vi "Process.vi"(0 "reference in":refnum<class "Grapher.lvclass">, 5 "error in":errorcluster) -> (14 "reference out":refnum<class "Grapher.lvclass">, 19 "error out":errorcluster)   [LabVIEW 2023, in "Grapher.lvclass"]
uses:
  Grapher.lvclass
  Grapher.lvclass/Grapher.ctl
  <vilib>/Utility/SystemLogging/NI_SystemLogging.lvlib
  Types/Indicators.ctl
  builds/PowerModuleInterface/PowerModuleInterface.lvlibp/Classes/PowerModule_interface/PowerModuleInterface.lvclass
panel:
  out "error info":errorcluster
  out "Last Command":string
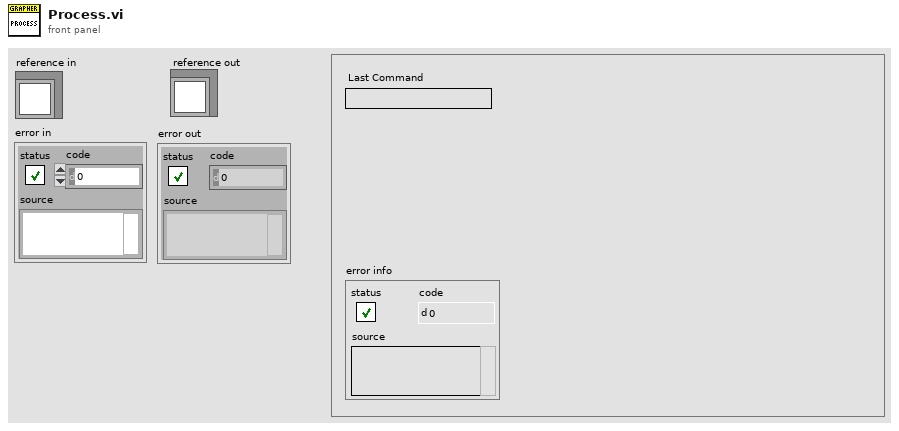
[diagram p1: front panel]
types:
  T1 = typedef "Indicators.ctl" = cluster{"XY Graph":refnum<vi>, "Mini Chart":refnum<vi>, "Voltage":refnum<vi>, "Current":refnum<vi>, "Power":refnum<vi>, "Function":refnum<vi>, "Charging":refnum<vi>, "Discharging":refnum<vi>}
  T2 = cluster{"Core":cluster{"Timeout":i32, "Events":cluster{"EventsToProcess":refnum<event-registration>}, "EventFromProcess":refnum<user-event>, "ProcessSyncQueue":refnum<queue>, "QueueFromProcess":refnum<queue>, "Command":string, "Data":variant}, "Chart History":cluster{"local timestamp":dbl[], "system timestamp":dbl[], "measured voltage":dbl[], "measured current":dbl[], "setpoint voltage":dbl[], "setpoint current":dbl[]}, "Use Local Time?":bool, "Graph Samples":u32, "Graph Decimation":i32, "Indicator Refs":T1, "Pause?":bool, "Power Module":refnum<class "PowerModuleInterface.lvclass">}
  T3 = cluster{"local timestamp":dbl[], "system timestamp":dbl[], "measured voltage":dbl[], "measured current":dbl[], "setpoint voltage":dbl[], "setpoint current":dbl[]}
  T4 = enum32{"Invalid", "Standard", "Closed", "Hidden", "Minimized", "Maximized"}
  T5 = cluster{"EventsToProcess":refnum<event-registration>}
  T6 = typedef "PowerModuleInterface.lvlibp/PowerModuleInterface.lvclass/Measurements.ctl" = cluster{"measured voltage (V)":dbl, "measured current (A)":dbl, "setpoint voltage (V)":dbl, "setpoint current (A)":dbl, "timestamp":dbl}
  T7 = typedef "Power Function.ctl" = enum16{"REGEN (LOAD)", "STANDBY", "SUPPLY (SOURCE)"}
  T8 = cluster{"system timestamp":dbl[], "measured voltage":dbl[]}
  T9 = cluster{"system timestamp":dbl[], "setpoint voltage":dbl[]}
  T10 = cluster{"system timestamp":dbl[], "measured current":dbl[]}
  T11 = cluster{"system timestamp":dbl[], "setpoint current":dbl[]}
  T12 = cluster{"system timestamp":dbl[], "setpoint current":dbl[]}[]
  T13 = typedef "Grapher.lvclass/ObjectAttributes.ctl" = cluster{"Indicator Refs":T1, "Update Rate (ms)":i32, "Power Module":refnum<class "PowerModuleInterface.lvclass">}
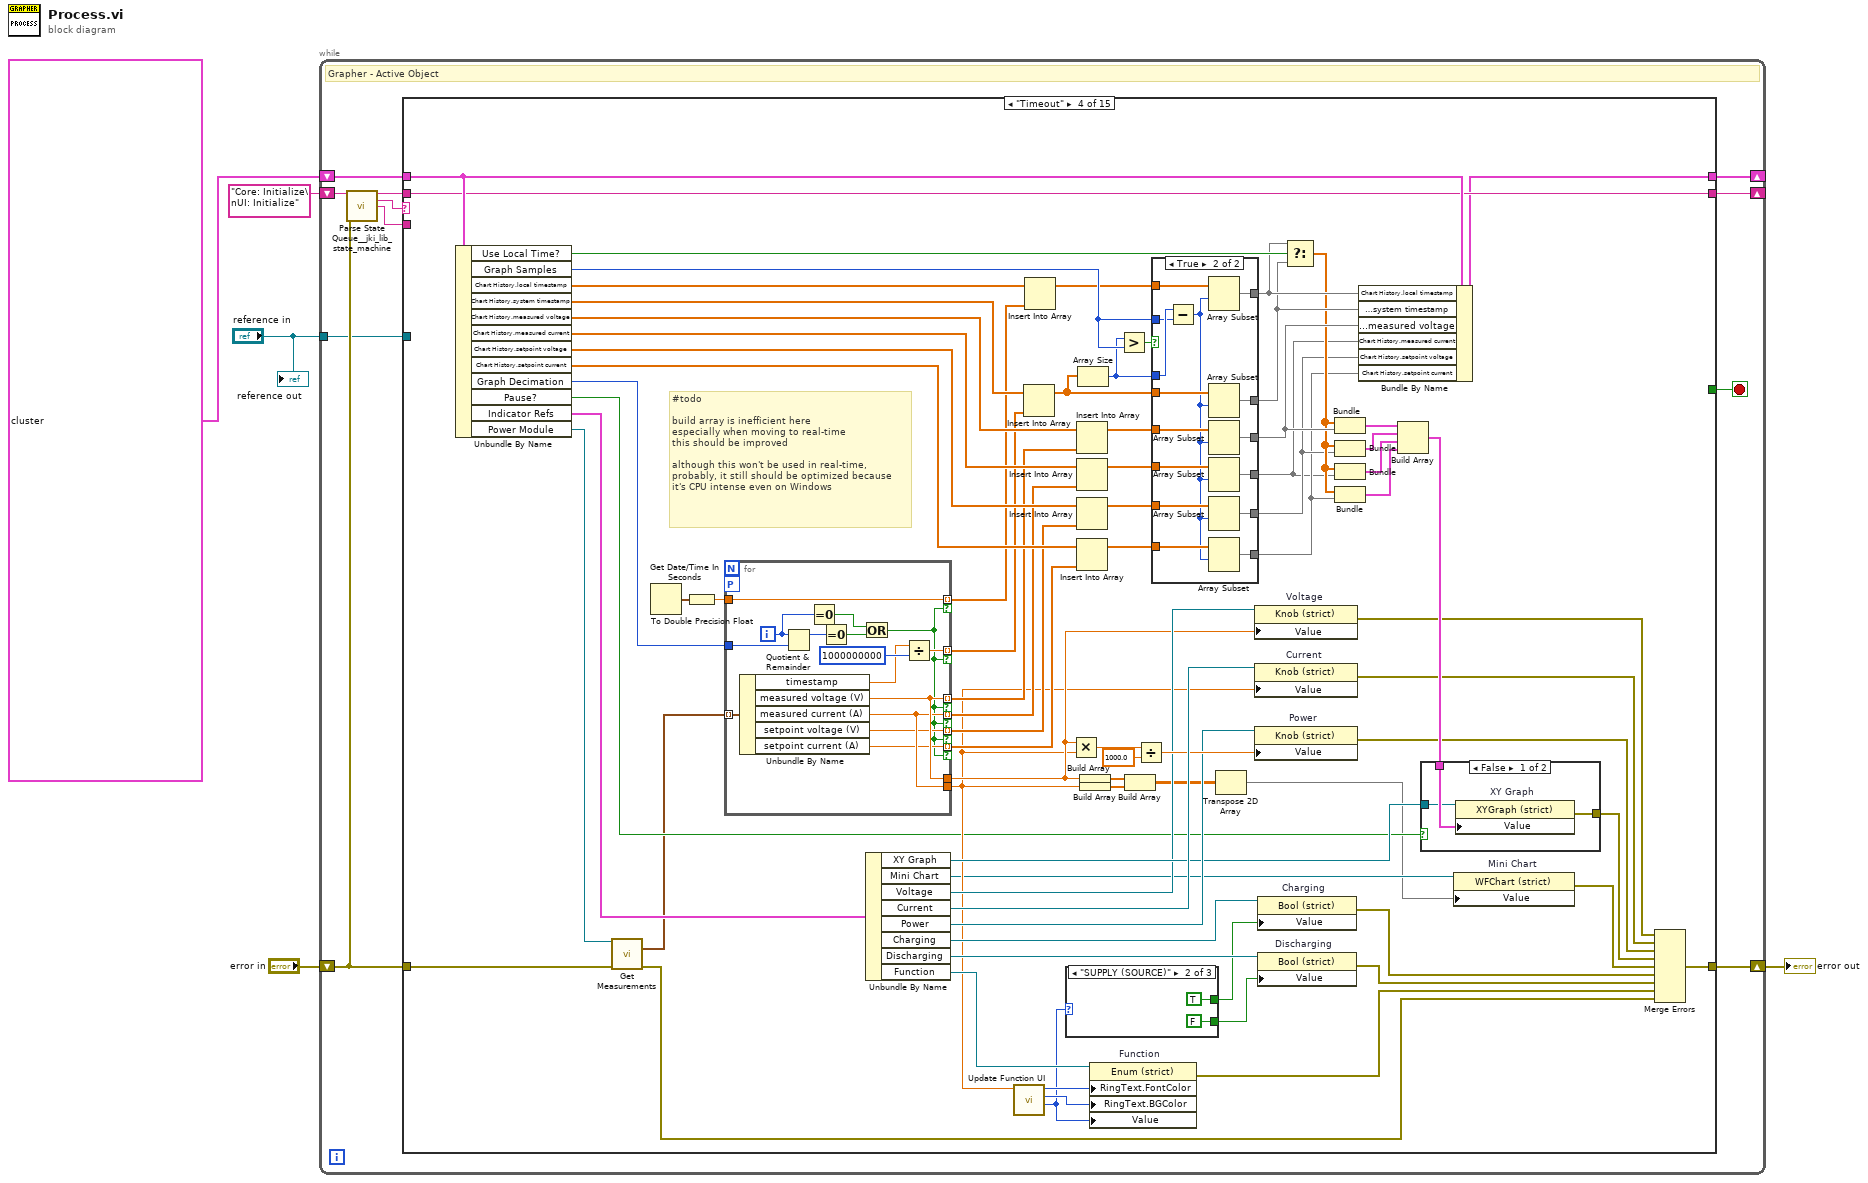
[diagram p0: block diagram]
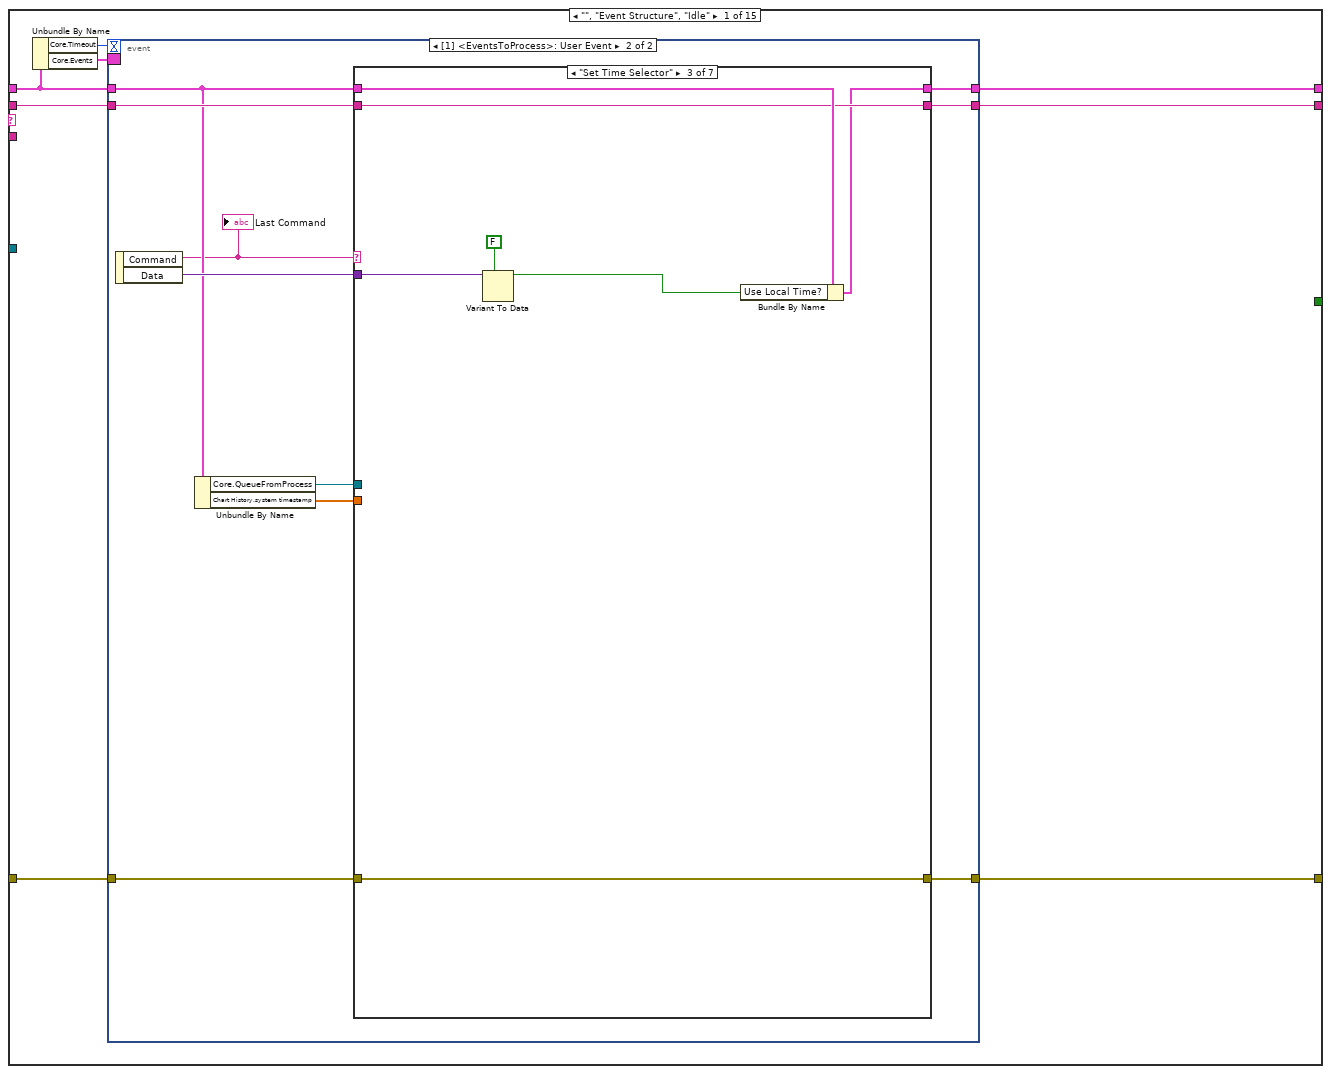
[diagram p2: hidden frame]
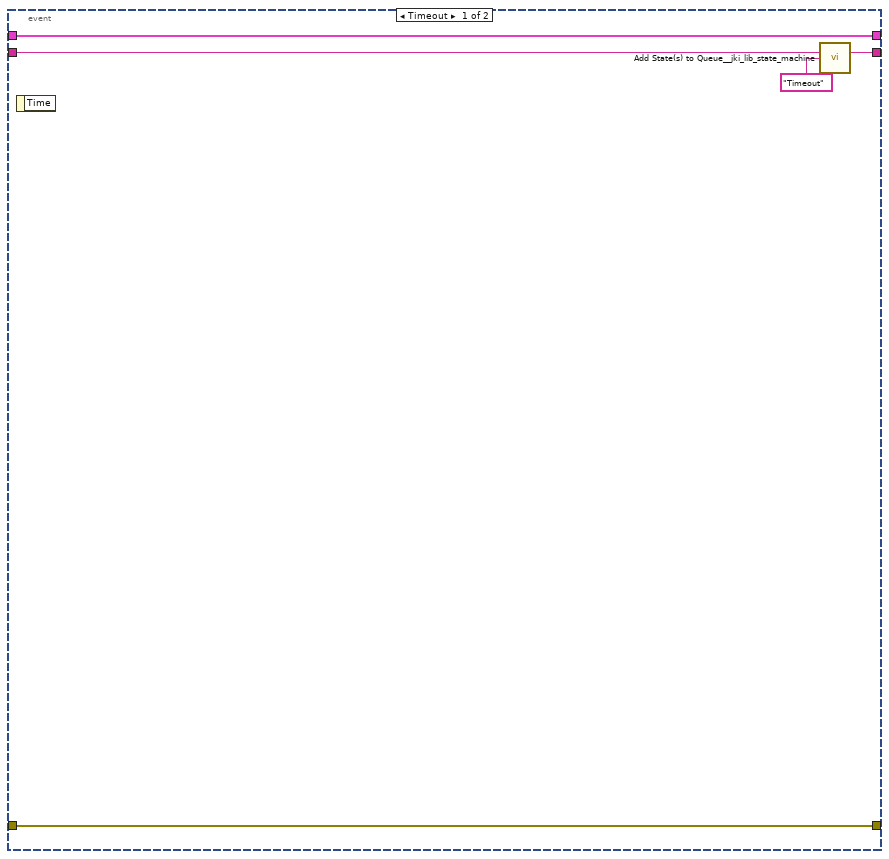
[diagram p3: hidden frame]
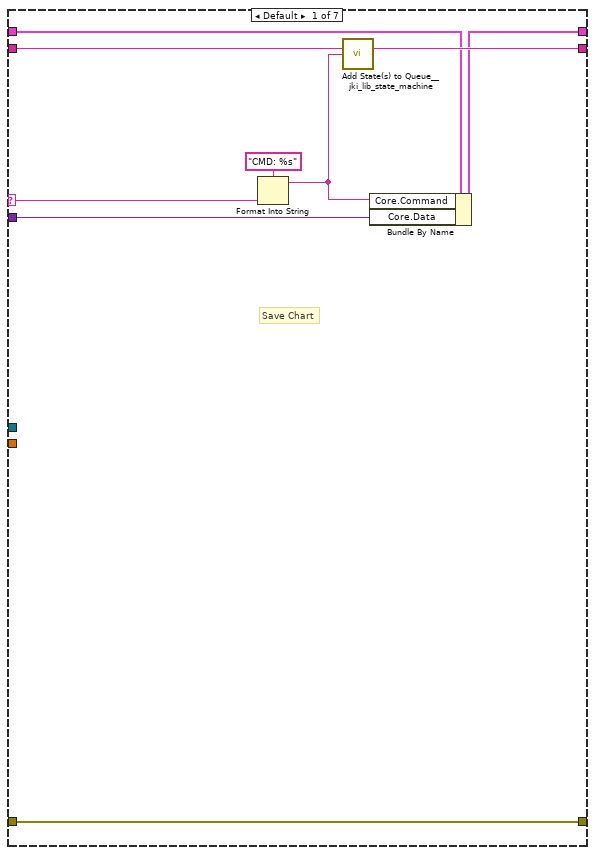
[diagram p4: hidden frame]
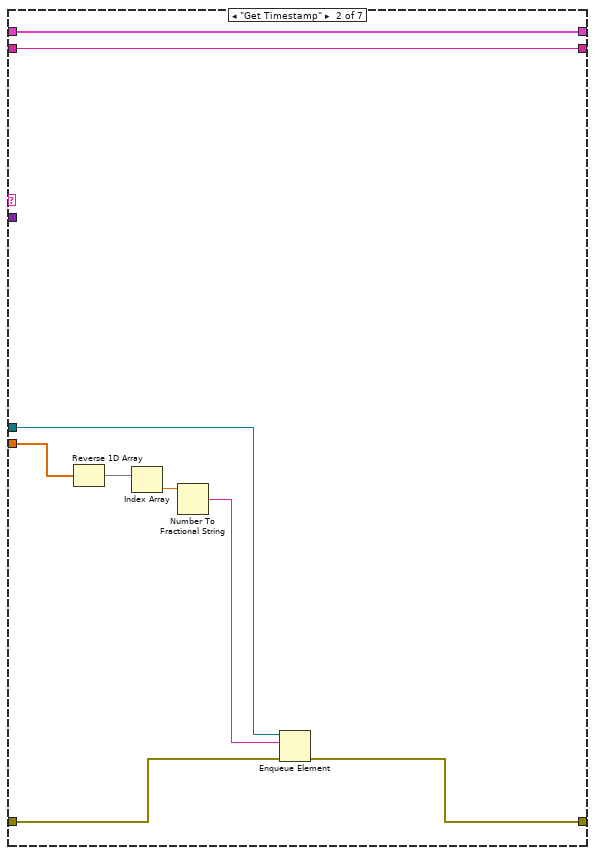
[diagram p5: hidden frame]
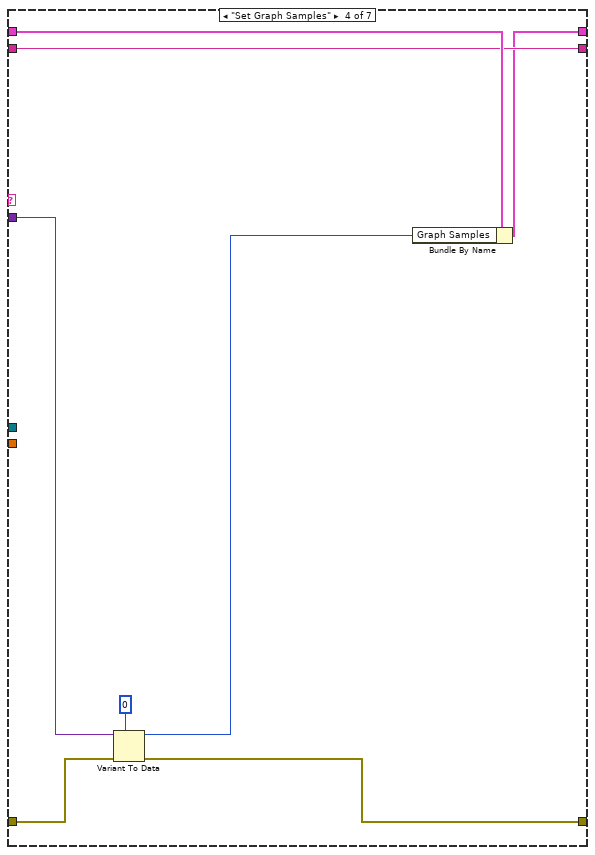
[diagram p6: hidden frame]
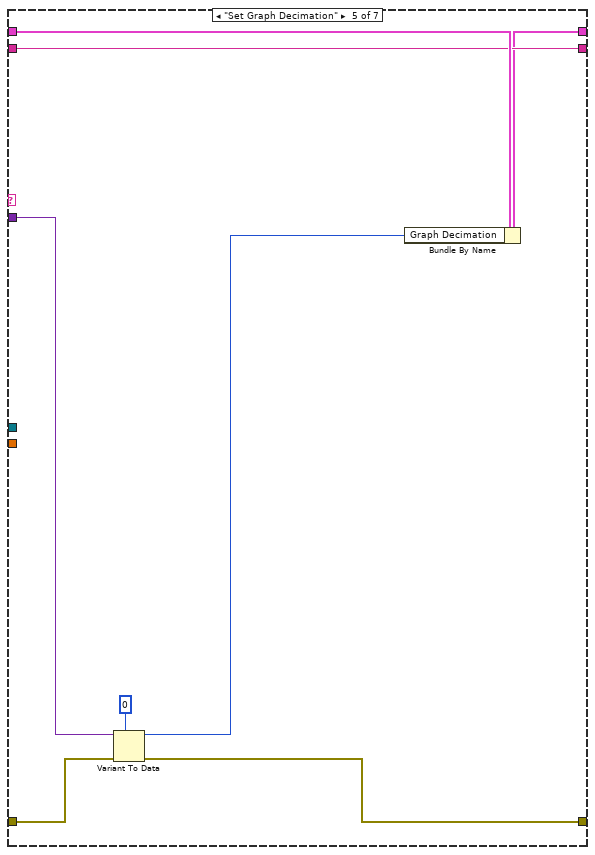
[diagram p7: hidden frame]
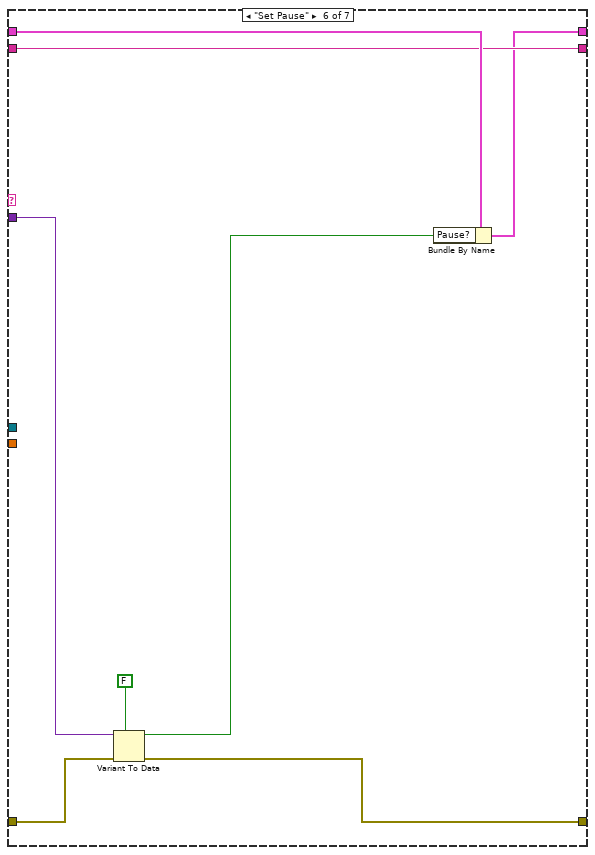
[diagram p8: hidden frame]
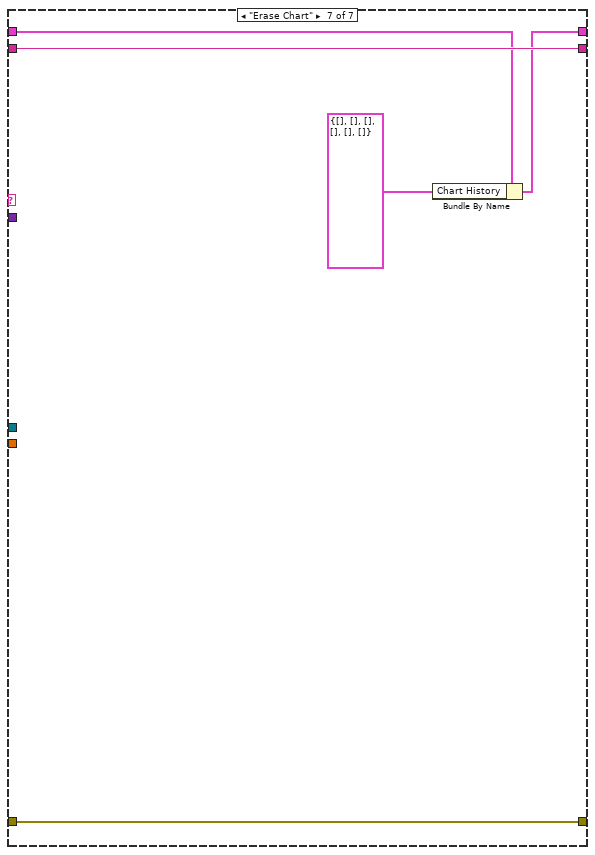
[diagram p9: hidden frame]
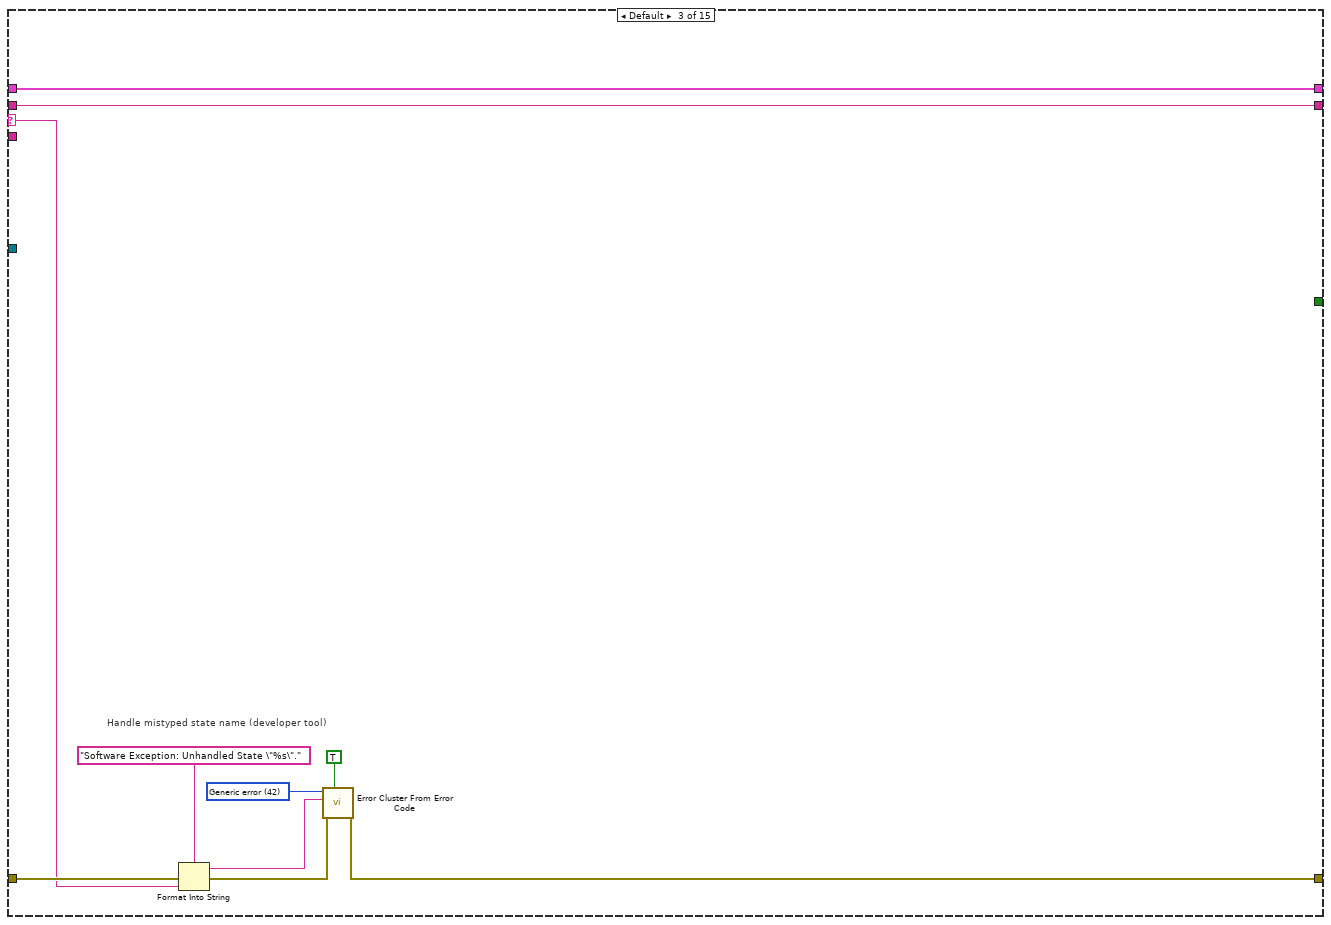
[diagram p11: hidden frame]
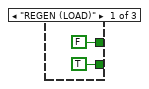
[diagram p12: hidden frame]
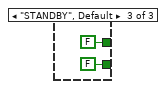
[diagram p13: hidden frame]
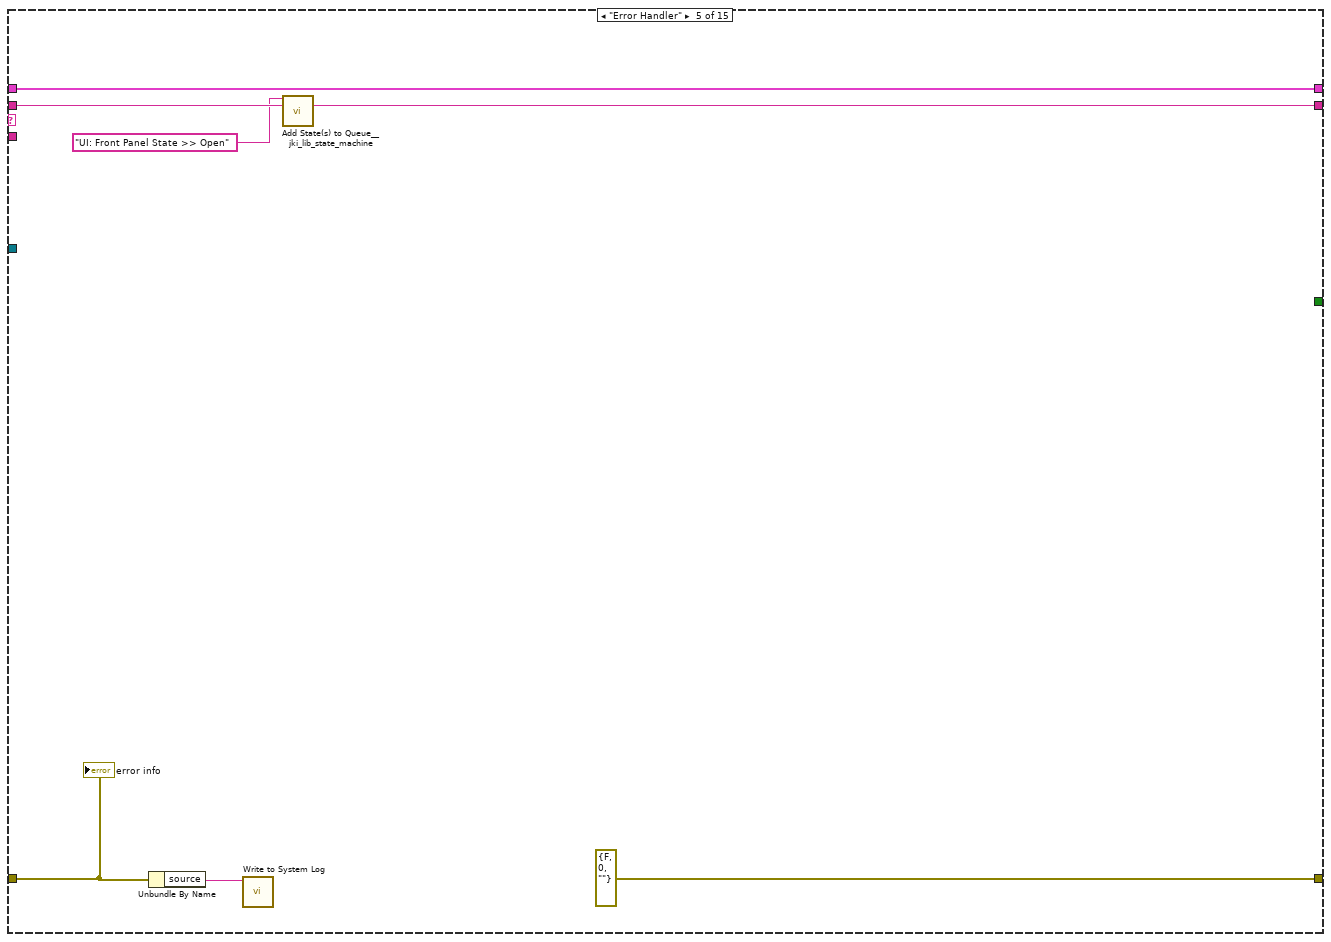
[diagram p16: hidden frame]
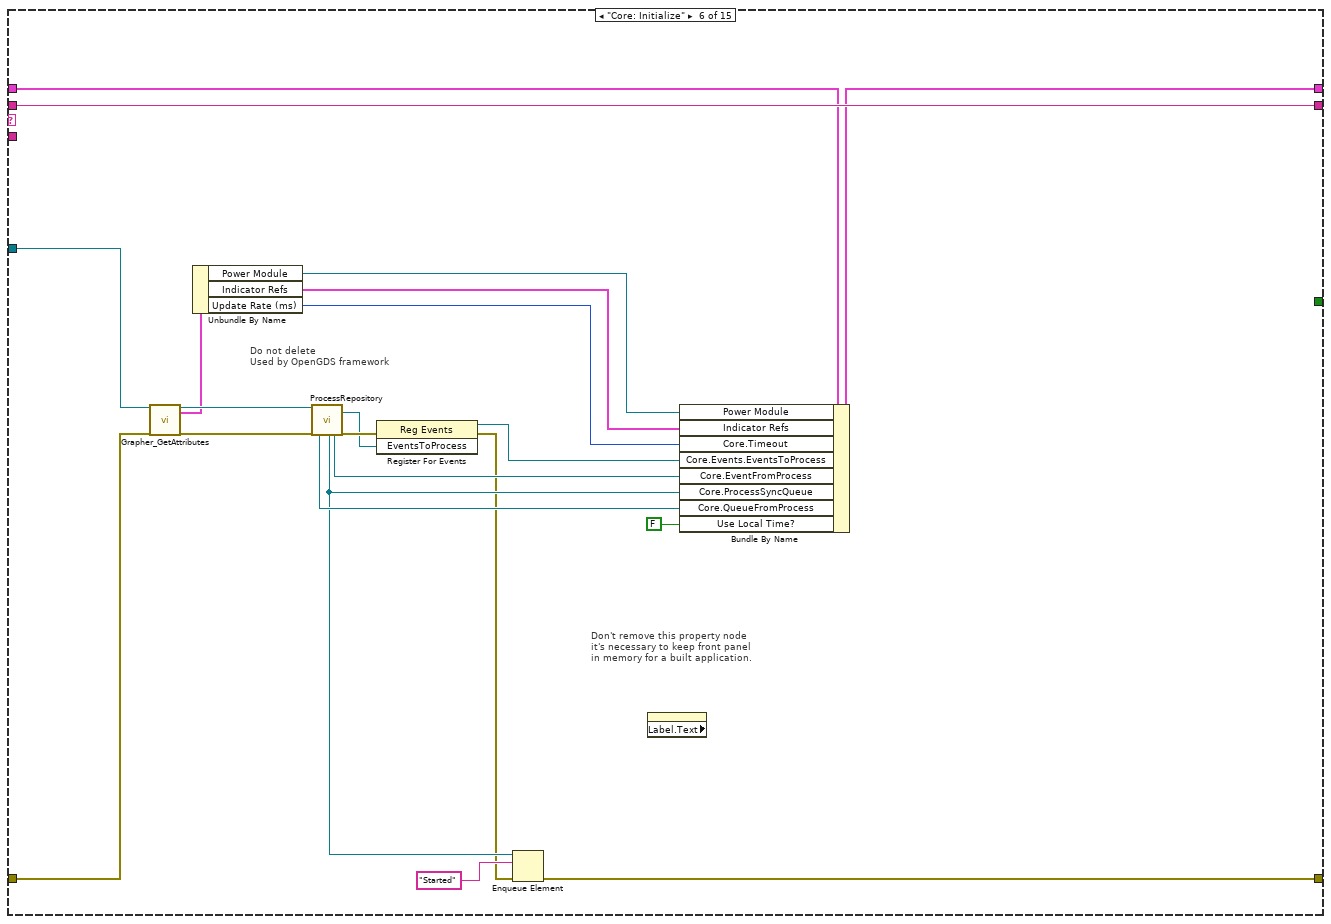
[diagram p17: hidden frame]
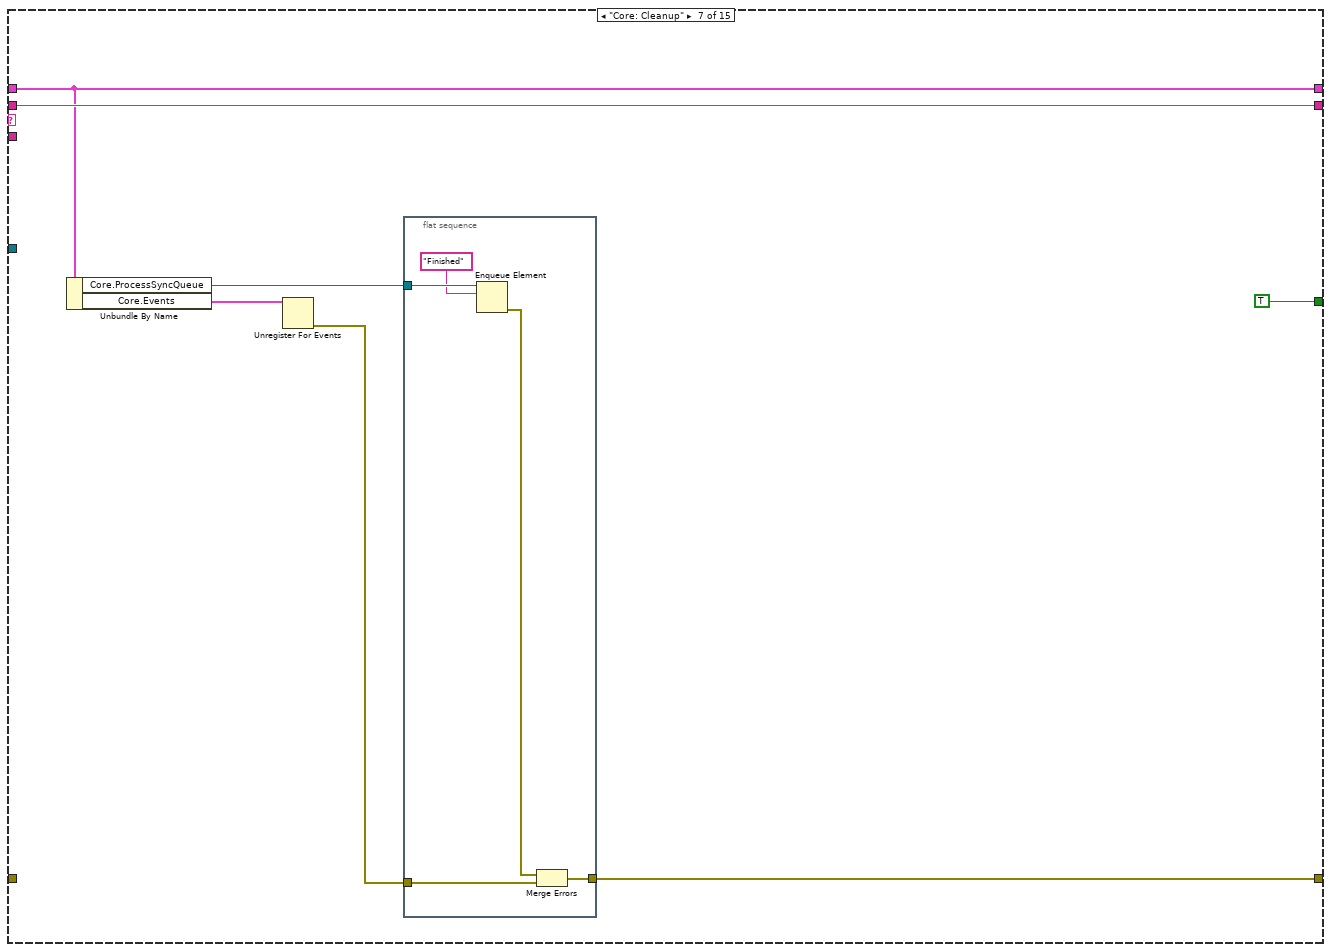
[diagram p18: hidden frame]
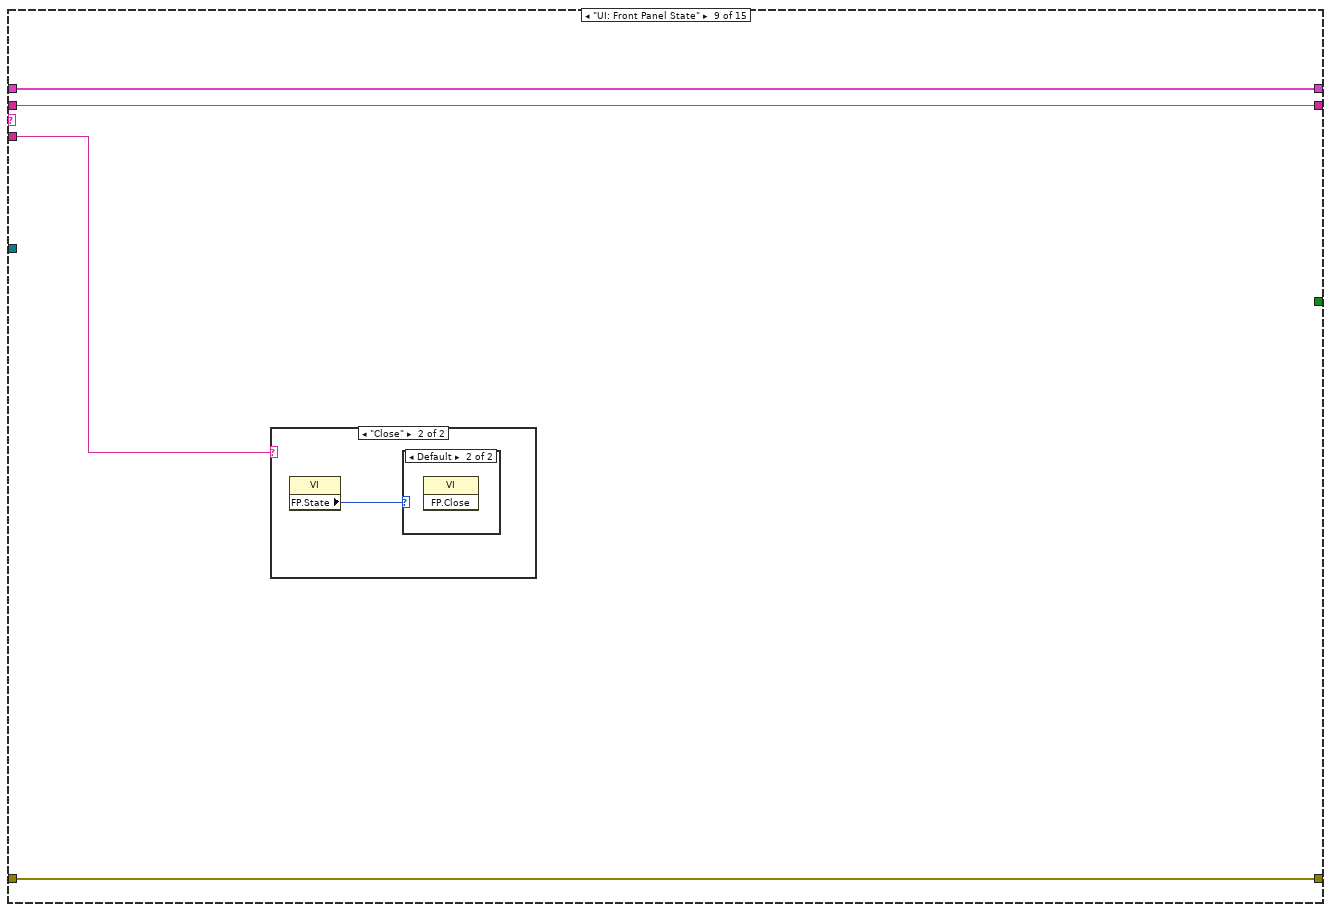
[diagram p20: hidden frame]
diagram:
  n1 = while {
    shift-right: [w15] -> w4
    shift-left: "error in" -> [w16]
    shift-right: [w8] -> _
    shift-left: "Core: Initialize\nUI: Initialize" ("States Out") -> [w11]
    shift-right: [w14] -> _
    shift-left: T2 {"Core"={"Timeout"=-1, "Events"={"EventsToProcess"=refnum}, "EventFromProcess"=refnum, "ProcessSyncQueue"=refnum, "QueueFromProcess"=refnum, "Command"="", "Data"=variant}, "Chart History"={"local timestamp"=[], "system timestamp"=[], "measured voltage"=[], "measured current"=[], "setpoint voltage"=[], "setpoint current"=[]}, "Use Local Time?"=FALSE, "Graph Samples"=1000, "Graph Decimation"=1000, "Indicator Refs"={"XY Graph"=refnum, "Mini Chart"=refnum, "Voltage"=refnum, "Current"=refnum, "Power"=refnum, "Function"=refnum, "Charging"=refnum, "Discharging"=refnum}, "Pause?"=FALSE, "Power Module"=refnum} ("LocalVariables") -> [w13]
    tunnel: "reference in" -> [w6]
    stop <- w7 stop-if-true
    # "Grapher - Active Object"
    n2 = call <vilib>:"Parse State Queue__jki_lib_state_machine.vi"("State Queue"=w11, "Error In (no error)"=w16) -> ("Remaining States"=w10:string, "Current State"=w12:string, "Arguments"=w9:string)  [unwired: 11 in]
    n3 = case shown="\"Timeout\"" w12 {
      selector: w12 -> [_ _ w97 _ _ _ _ _ _ _ _ _ _ _ _]
      tunnel: w16 -> [w18 w96 w99 w114 w231 w244 _ w271 w272 w295 _ w302 w305 w312 w314]
      tunnel: [w19 w96 w98 w182 errorcluster {"status"=FALSE, "code"=0, "source"=""} ("error constant") w256 w259 w271 w272 w295 w296 w302 w305 w312 w313] -> w15
      tunnel: [w24 w95 w106 w180 w235 w254 w260 w270 w274 w287 w297 w301 w304 w311 w316] -> w14
      tunnel: w13 -> [w20 w95 w106 w183 w235 w253 w260 w270 w274 w287 w297 w301 w304 w311 w316]
      tunnel: w10 -> [w22 w94 w105 w181 w234 w255 w263 w269 w275 w294 w299 w300 _ w310 w317]
      tunnel: w9 -> [_ _ _ _ _ _ _ _ w273 _ _ _ _ w307 _]
      tunnel: [w21 w94 w105 w181 w233 w255 w263 w269 w275 w294 w299 w300 "UI: Cleanup\nCore: Cleanup" ("State(s) at Back (\"\")") w309 w317] -> w8
      tunnel: [_ _ _ _ _ _ TRUE _ _ _ _ _ _ _ _] -> w7
      tunnel: w6 -> [_ _ _ _ _ w242 _ _ _ _ _ _ _ _ _]
      frame "", "Event Structure", "Idle" {
        n4 = Unbundle By Name(w20) -> ("Core.Timeout"=w17:i32, "Core.Events"=w23:T5)
        n5 = event shown="[1] <EventsToProcess>: User Event" {
          selector: w23 -> [_ _]
          dyn-events: _ -> [_ _]
          timeout: w17 -> [_ _]
          tunnel: w20 -> [w29 w34]
          tunnel: [w29 w37] -> w24
          tunnel: [w27 w39] -> w21
          tunnel: w22 -> [w28 w38]
          tunnel: [w25 w30] -> w19
          tunnel: w18 -> [w25 w31]
          event Timeout {
            n6 = event-data() -> ()  [unwired: 1 in, 1 out]
            n7 = call <vilib>:"Add State(s) to Queue__jki_lib_state_machine.vi"("State(s) in (\"\")"=w28, "State(s) at Back (\"\")"="Timeout" ("State(s) at Back (\"\")")) -> ("States Out"=w27:string)  [unwired: 13 in]
          }
          event User Event {
            n8 = event-data() -> ("Command"=w33:string, "Data"=w36:variant)  [unwired: 1 in]
            "Last Command" <- w33
            n9 = Unbundle By Name(w34) -> ("Core.QueueFromProcess"=w35:refnum<queue>, "Chart History.system timestamp"=w32:dbl[])
            n10 = case shown="\"Set Time Selector\"" w33 {
              selector: w33 -> [w41 _ _ _ _ _ _]
              tunnel: [w48 w55 w62 w69 w77 w85 w93] -> w39
              tunnel: w38 -> [w47 w55 w62 w69 w77 w85 w93]
              tunnel: [w46 w56 w59 w68 w76 w84 w91] -> w37
              tunnel: w36 -> [w45 _ w64 w71 w79 w87 _]
              tunnel: w35 -> [_ w57 _ _ _ _ _]
              tunnel: w34 -> [w44 w56 w63 w70 w78 w86 w92]
              tunnel: w32 -> [_ w53 _ _ _ _ _]
              tunnel: w31 -> [w40 w54 w58 w72 w80 w88 w90]
              tunnel: [w40 w49 w58 w67 w75 w83 w90] -> w30
              frame Default {
                # "Save Chart"
                n11 = Format Into String(format string="CMD: %s", w41) -> (resulting string=w42:string)  [unwired: 2 in, 1 out]
                n12 = call <vilib>:"Add State(s) to Queue__jki_lib_state_machine.vi"("State(s) in (\"\")"=w47, "State(s) at Back (\"\")"=w42) -> ("States Out"=w48:string)  [unwired: 13 in]
                n13 = Bundle By Name(cluster=w44, "Core.Command"=w42, "Core.Data"=w45) -> (w46:T2)
              }
              frame "Get Timestamp" {
                n14 = Reverse 1D Array(array=w53) -> (reversed array=w52:dbl[])
                n15 = Index Array(array=w52) -> (element=w51:dbl)  [unwired: 1 in]
                n16 = Number To Fractional String(number=w51) -> (F-format string=w50:string)  [unwired: 3 in]
                n17 = Enqueue Element ("Return message to the client from this process")(queue=w57, element=w50, error in (no error)=w54) -> (error out=w49:errorcluster)  [unwired: 1 in, 2 out]
              }
              frame "Set Time Selector" {
                n18 = Variant To Data(type=FALSE, Variant=w64) -> (data=w61:bool)  [unwired: 1 in, 1 out]
                n19 = Bundle By Name(cluster=w63, "Use Local Time?"=w61) -> (w59:T2)
              }
              frame "Set Graph Samples" {
                n20 = Variant To Data(error in=w72, type=u32 0 ("Graph Samples"), Variant=w71) -> (data=w65:u32, error out=w67:errorcluster)
                n21 = Bundle By Name(cluster=w70, "Graph Samples"=w65) -> (w68:T2)
              }
              frame "Set Graph Decimation" {
                n22 = Variant To Data(error in=w80, type=0 ("Graph Samples"), Variant=w79) -> (data=w73:i32, error out=w75:errorcluster)
                n23 = Bundle By Name(cluster=w78, "Graph Decimation"=w73) -> (w76:T2)
              }
              frame "Set Pause" {
                n24 = Variant To Data(error in=w88, type=FALSE, Variant=w87) -> (data=w82:bool, error out=w83:errorcluster)
                n25 = Bundle By Name(cluster=w86, "Pause?"=w82) -> (w84:T2)
              }
              frame "Erase Chart" {
                n26 = Bundle By Name(cluster=w92, "Chart History"=T3 {"local timestamp"=[], "system timestamp"=[], "measured voltage"=[], "measured current"=[], "setpoint voltage"=[], "setpoint current"=[]}) -> (w91:T2)
              }
            }
          }
        }
      }
      frame "---------- Core ----------" {
      }
      frame Default {
        w103 = 42 items=["No error", "Argument error", "Memory is full", "Out of zone", "End of file", "File already open", "Generic file I/O error", "File not found", "File permission error", "Disk is full", "Duplicate path", "Too many files open", "System feature not enabled", "Resource file not found", "Cannot add resource", "Resource not found", "Image not found", "Image memory error", "Pen does not exist", "Config type invalid", "Config token not found", "Config parse error", "Config memory error", "Bad external code format", "Bad external code offset", "External code not present", "Null window", "Destroy window error", "Null menu", "Print aborted", "Bad print record", "Print driver error", "Windows error during printing", "Memory error during printing", "Print dialog error", "Generic print error", "Invalid device refnum", "Device not found", "Device parameter error", "Device unit error", "Cannot open device", "Device call aborted", "Generic error", "Cancelled by user", "Object ID too low", "Object ID too high", "Object not in heap", "Unknown heap", "Unknown object (invalid DefProc)", "Unknown object (DefProc not in table)", "Message out of range", "Invalid (null) method", "Unknown message", "Manager call not supported", "Bad address", "Network operation in progress", "Network operation timed out", "Connection is busy", "Network attribute not supported", "Network error", "Address in use", "System out of memory", "Connection aborted", "Connection refused", "Not connected", "Already connected", "Connection closed", "Initialization error (interapplication manager)", "Bad occurrence", "Wait on unbound occurrence handler", "Occurrence queue overflow", "Datalog type conflict", "Unused", "Unrecognized type (interapplication manager)", "Memory corrupt", "Failed to make temporary DLL", "Old CIN version", "Drag socket not found", "Failed to load drop-object", "Failed to register OLE object", "Failed to release OLE object", "Format specifier type mismatch", "Unknown format specifier", "Too few format specifiers", "Too many format specifiers", "Scan failed", "Newer CIN version", "Error converting to variant", "Runtime menu error", "Password tampered", "Variant attribute not found", "Incompatible variant data type", "Event data is not available", "Event Store is not present", "Occurrence is not found", "Event Queue is not created", "Event info is not available", "Refnum passed is NULL", "Error retrieving Class GUID", "Error retrieving CoClass GUID", "Error retrieving TypeLib GUID.", "Bad built application magic bytes.", "Specific driver is different from the specific driver associated with the Logical Name.", "There is no session opened to the class driver.", "Max Error", "MAX - Error with config objects", "MAX - Error loading configuration", "MAX - Group not supported"]
        # "Handle mistyped state name (developer tool)"
        n27 = Format Into String(format string="Software Exception: Unhandled State \"%s\"." ("message"), error in=w99, w97) -> (resulting string=w102:string, error out=w101:errorcluster)  [unwired: 1 in]
        n28 = call <vilib>:"Error Cluster From Error Code.vi"("show call chain? (False)"=TRUE, "error in (no error)"=w101, "error message (\"\")"=w102, "error code (0)"=w103) -> ("error out"=w98:errorcluster)  [unwired: 5 in]
      }
      frame "Timeout" {
        # "#todo\n\nbuild array is inefficient here\nespecially when moving to real-time\nthis should be improved\n\nalthough this won't be used in real-time,\nprobably, it still should be optimized because\nit's CPU intense even on Windows"
        n29 = Unbundle By Name(w183) -> ("Use Local Time?"=w171:bool, "Graph Samples"=w179:u32, "Chart History.local timestamp"=w178:dbl[], "Chart History.system timestamp"=w177:dbl[], "Chart History.measured voltage"=w176:dbl[], "Chart History.measured current"=w175:dbl[], "Chart History.setpoint voltage"=w174:dbl[], "Chart History.setpoint current"=w173:dbl[], "Graph Decimation"=w172:i32, "Pause?"=w110:bool, "Indicator Refs"=w111:T1, "Power Module"=w112:refnum<class "PowerModuleInterface.lvclass">)
        n30 = call-dynamic "Get Measurements.vi"("object in"=w112, "Error In"=w114) -> ("measurements"=w109:T6[], "Error Out"=w113:errorcluster)  [unwired: 11 in, 1 out]
        n31 = Get Date/Time In Seconds() -> (seconds since 1Jan1904=w163:timestamp)
        n32 = To Double Precision Float(number=w163) -> (double precision float=w143:dbl)
        n33 = for {
          tunnel: w109 -> [w207] mode=indexing
          tunnel: [w205] -> w144 mode=indexing if=w193
          tunnel: [w204] -> w145 mode=indexing if=w193
          tunnel: [w202] -> w154 mode=indexing if=w193
          tunnel: [w201] -> w153 mode=indexing if=w193
          tunnel: [w203] -> w149 mode=indexing if=w193
          workers-P: _ -> [_]
          tunnel: [w205] -> w119
          tunnel: [w204] -> w118
          tunnel: w172 -> [w199]
          tunnel: w143 -> [w194]
          tunnel: [w194] -> w142 mode=indexing if=w193
          i -> [w196]
          n34 = Unbundle By Name(w207) -> ("timestamp"=w200:dbl, "measured voltage (V)"=w205:dbl, "measured current (A)"=w204:dbl, "setpoint voltage (V)"=w203:dbl, "setpoint current (A)"=w202:dbl)
          n35 = Quotient & Remainder(x=w196, y=w199) -> (x-y*floor(x/y)=w198:i32)  [unwired: 1 out]
          n36 = Equal To 0?(x=w196) -> (x = 0?=w195:bool)
          n37 = Equal To 0?(x=w198) -> (x = 0?=w197:bool)
          n38 = Or(x=w195, y=w197) -> (x .or. y?=w193:bool)
          n39 = Divide(x=w200, y=i64 1000000000) -> (x/y=w201:dbl)
        }
        n40 = Unbundle By Name(w111) -> ("XY Graph"=w129:refnum<vi>, "Mini Chart"=w115:refnum<vi>, "Voltage"=w120:refnum<vi>, "Current"=w138:refnum<vi>, "Power"=w136:refnum<vi>, "Charging"=w128:refnum<vi>, "Discharging"=w130:refnum<vi>, "Function"=w131:refnum<vi>)
        n41 = call "Update Function UI.vi"("measured_current"=w118) -> ("Function"=w126:T7, "BG Color"=w140:u32, "Font Color"=w141:u32)  [unwired: 8 in]
        n42 = Insert Into Array(array=w177, new element=w153) -> (w151:dbl[])  [unwired: 1 in]
        n43 = Insert Into Array(array=w178, new element=w142) -> (w152:dbl[])  [unwired: 1 in]
        n44 = case shown="\"SUPPLY (SOURCE)\"" w126 {
          tunnel: [TRUE FALSE FALSE] -> w125
          tunnel: [FALSE TRUE FALSE] -> w124
          frame "REGEN (LOAD)" {
          }
          frame "SUPPLY (SOURCE)" {
          }
          frame "STANDBY", Default {
          }
        }
        n45 = Multiply(x=w119, y=w118) -> (x*y=w170:dbl)
        n46 = Insert Into Array(array=w176, new element=w144) -> (w158:dbl[])  [unwired: 1 in]
        n47 = Insert Into Array(array=w175, new element=w145) -> (w157:dbl[])  [unwired: 1 in]
        n48 = Insert Into Array(array=w174, new element=w149) -> (w156:dbl[])  [unwired: 1 in]
        n49 = Insert Into Array(array=w173, new element=w154) -> (w155:dbl[])  [unwired: 1 in]
        n50 = Array Size(array=w151) -> (size(s)=w150:i32)
        n51 = Build Array(w119) -> (w117:dbl[])
        n52 = Build Array(w118) -> (w116:dbl[])
        n53 = property on="Function" class="Enum (strict)"(reference=w131, "RingText.FontColor"=w141, "RingText.BGColor"=w140, "Value"=w126) -> (error out=w127:errorcluster)  [unwired: 1 in, 1 out]
        n54 = Greater?(x=w150, y=w179) -> (0:w159:bool)
        n55 = Build Array(w117, w116) -> (w108:dbl[][])
        n56 = Divide(x=w170, y=1000.0) -> (x/y=w137:dbl)
        n57 = case shown="True" w159 {
          tunnel: w151 -> [w213 w224]
          tunnel: w158 -> [w212 w222]
          tunnel: w157 -> [w211 w220]
          tunnel: w156 -> [w210 w218]
          tunnel: w155 -> [w209 w217]
          tunnel: [w209 w216] -> w147
          tunnel: [w210 w215] -> w148
          tunnel: [w211 w219] -> w146
          tunnel: [w212 w221] -> w164
          tunnel: [w213 w223] -> w161
          tunnel: w152 -> [w208 w226]
          tunnel: [w208 w225] -> w162
          tunnel: w150 -> [_ w228]
          tunnel: w179 -> [_ w227]
          frame False {
          }
          frame True {
            n58 = Subtract(x=w228, y=w227) -> (x-y=w214:u32)
            n59 = Array Subset(array=w226, index=w214) -> (w225:dbl[])  [unwired: 1 in]
            n60 = Array Subset(array=w224, index=w214) -> (w223:dbl[])  [unwired: 1 in]
            n61 = Array Subset(array=w222, index=w214) -> (w221:dbl[])  [unwired: 1 in]
            n62 = Array Subset(array=w220, index=w214) -> (w219:dbl[])  [unwired: 1 in]
            n63 = Array Subset(array=w218, index=w214) -> (w215:dbl[])  [unwired: 1 in]
            n64 = Array Subset(array=w217, index=w214) -> (w216:dbl[])  [unwired: 1 in]
          }
        }
        n65 = Transpose 2D Array(2D array=w108) -> (transposed array=w107:dbl[][])
        n66 = property on="Voltage" class="Knob (strict)"(reference=w120, "Value"=w119) -> (error out=w132:errorcluster)  [unwired: 1 in, 1 out]
        n67 = property on="Current" class="Knob (strict)"(reference=w138, "Value"=w118) -> (error out=w133:errorcluster)  [unwired: 1 in, 1 out]
        n68 = property on="Power" class="Knob (strict)"(reference=w136, "Value"=w137) -> (error out=w134:errorcluster)  [unwired: 1 in, 1 out]
        n69 = property on="Charging" class="Bool (strict)"(reference=w128, "Value"=w124) -> (error out=w122:errorcluster)  [unwired: 1 in, 1 out]
        n70 = property on="Discharging" class="Bool (strict)"(reference=w130, "Value"=w125) -> (error out=w123:errorcluster)  [unwired: 1 in, 1 out]
        n71 = Select(t=w162, s=w171, f=w161) -> (s? t:f=w160:dbl[])
        n72 = Bundle("system timestamp"=w160, "measured voltage"=w164) -> (w168:T8)  [unwired: 1 in]
        n73 = Bundle("system timestamp"=w160, "setpoint voltage"=w148) -> (w167:T9)  [unwired: 1 in]
        n74 = Bundle("system timestamp"=w160, "measured current"=w146) -> (w166:T10)  [unwired: 1 in]
        n75 = Bundle("system timestamp"=w160, "setpoint current"=w147) -> (w165:T11)  [unwired: 1 in]
        n76 = Bundle By Name(cluster=w183, "Chart History.local timestamp"=w162, "Chart History.system timestamp"=w161, "Chart History.measured voltage"=w164, "Chart History.measured current"=w146, "Chart History.setpoint voltage"=w148, "Chart History.setpoint current"=w147) -> (w180:T2)
        n77 = Build Array(w168, w167, w166, w165) -> (w139:T12)
        n78 = case shown="False" w110 {
          tunnel: w139 -> [w192 _]
          tunnel: w129 -> [w191 _]
          tunnel: [w190 _] -> w135
          frame False {
            n79 = property on="XY Graph" class="XYGraph (strict)"(reference=w191, "Value"=w192) -> (error out=w190:errorcluster)  [unwired: 1 in, 1 out]
          }
          frame True {
          }
        }
        n80 = property on="Mini Chart" class="WFChart (strict)"(reference=w115, "Value"=w107) -> (error out=w121:errorcluster)  [unwired: 1 in, 1 out]
        n81 = Merge Errors(w132, w133, w134, w135, w121, w122, w123, w127, w113) -> (w182:errorcluster)
      }
      frame "Error Handler" {
        n82 = Unbundle By Name(w231) -> ("source"=w229:string)
        n83 = call <vilib>:"Write to System Log.vi"("message"=w229) -> ()  [unwired: 10 in, 1 out]
        n84 = call <vilib>:"Add State(s) to Queue__jki_lib_state_machine.vi"("State(s) in Front (\"\")"="UI: Front Panel State >> Open" ("State(s) at Back (\"\")"), "State(s) in (\"\")"=w234) -> ("States Out"=w233:string)  [unwired: 13 in]
        "error info" <- w231
      }
      frame "Core: Initialize" {
        # "Do not delete\nUsed by OpenGDS framework"
        # "Don't remove this property node\nit's necessary to keep front panel\nin memory for a built application."
        # "Template created by VI Technologies"
        n85 = call "Grapher_GetAttributes.vi"("reference in"=w242, "Error In"=w244) -> ("reference out"=w241:refnum<class "Grapher.lvclass">, "Data"=w240:T13, "Error Out"=w243:errorcluster)  [unwired: 14 in, 1 out]
        n86 = Unbundle By Name(w240) -> ("Power Module"=w236:refnum<class "PowerModuleInterface.lvclass">, "Indicator Refs"=w238:T1, "Update Rate (ms)"=w239:i32)
        n87 = call "ProcessRepository.vi"("reference in"=w241, "Error In"=w243) -> ("QueueFromProcess"=w248:refnum<queue>, "ProcessSyncQueue"=w246:refnum<queue>, "EventFromProcess"=w249:refnum<user-event>, "EventsToProcess"=w251:refnum<user-event>, "Error Out"=w252:errorcluster)  [unwired: 10 in, 3 out]
        n88 = register-events(error in=w252, w251) -> (reference out=w250:refnum<event-registration>, error out=w245:errorcluster)  [unwired: 1 in]
        n89 = Enqueue Element(queue=w246, element="Started", error in (no error)=w245) -> (error out=w256:errorcluster)  [unwired: 1 in, 2 out]
        n90 = property on="reference in" class="LVClassControl (strict)" props=["Label", "Text"]() -> ()  [unwired: 2 in, 3 out]
        n91 = Bundle By Name(cluster=w253, "Power Module"=w236, "Indicator Refs"=w238, "Core.Timeout"=w239, "Core.Events.EventsToProcess"=w250, "Core.EventFromProcess"=w249, "Core.ProcessSyncQueue"=w246, "Core.QueueFromProcess"=w248, "Use Local Time?"=FALSE ("Connected?")) -> (w254:T2)
      }
      frame "Core: Cleanup" {
        n92 = Unbundle By Name(w260) -> ("Core.ProcessSyncQueue"=w261:refnum<queue>, "Core.Events"=w258:T5)
        n93 = Unregister For Events(event registration refnum=w258) -> (error out=w257:errorcluster)  [unwired: 1 in]
        n94 = flat-sequence {
          tunnel: [w267] -> w259
          tunnel: w261 -> [w266]
          tunnel: w257 -> [w265]
          frame #0 {
            n95 = Enqueue Element(queue=w266, element="Finished") -> (error out=w268:errorcluster)  [unwired: 2 in, 2 out]
            n96 = Merge Errors(w268, w265) -> (w267:errorcluster)
          }
        }
      }
      frame "---------- UI ----------" {
      }
      frame "UI: Front Panel State" {
        n97 = case shown="\"Close\"" w273 {
          frame "Open", Default {
            n98 = property class="VI"() -> ("FP.State"=w276:T4)  [unwired: 2 in, 2 out]
            n99 = case shown="Default" w276 {
              frame Default {
                n100 = invoke class="VI" method="FP.Open"("Activate"=TRUE, "State"=T4."Standard") -> ()  [unwired: 3 in, 5 out]
              }
              frame "Standard" {
              }
            }
          }
          frame "Close" {
            n101 = property class="VI"() -> ("FP.State"=w279:T4)  [unwired: 2 in, 2 out]
            n102 = case shown="Default" w279 {
              frame "Closed" {
              }
              frame Default {
                n103 = invoke class="VI" method="FP.Close"() -> ()  [unwired: 3 in, 3 out]
              }
            }
          }
        }
      }
      frame "UI: Initialize" {
        n104 = property class="VI"() -> ("Name"=w293:string)  [unwired: 2 in, 2 out]
        n105 = Match Pattern(string=w293, regular expression="\\2Evi$") -> (before substring=w291:string)  [unwired: 1 in, 3 out]
        n106 = Reverse String(1:w291) -> (0:w290:string)
        n107 = Match Pattern(string=w290, regular expression=":") -> (before substring=w288:string, after substring=w286:string)  [unwired: 1 in, 2 out]
        n108 = Match Pattern(string=w286, regular expression="\\2E") -> (after substring=w284:string)  [unwired: 1 in, 3 out]
        n109 = Reverse String(1:w284) -> (0:w283:string)
        n110 = Reverse String(1:w288) -> (0:w282:string)
        n111 = Format Into String(format string="%s %s", w283, w282) -> (resulting string=w281:string)  [unwired: 2 in, 1 out]
        n112 = property class="VI"("Front Panel.Title"=w281) -> ()  [unwired: 2 in, 2 out]
      }
      frame "UI: Cleanup" {
        n113 = property class="VI"() -> (error out=w296:errorcluster, "FP.State"=w298:T4)  [unwired: 2 in, 1 out]
        n114 = case shown="\"Standard\", Default" w298 {
          frame "Closed" {
          }
          frame "Standard", Default {
            n115 = invoke class="VI" method="FP.Close"() -> ()  [unwired: 3 in, 3 out]
          }
        }
      }
      frame "---------- CMD ----------" {
      }
      frame "CMD: Exit" {
      }
      frame "CMD: Front Panel State" {
        n116 = Format Into String(format string="UI: Front Panel State>>%s" ("string"), w307) -> (resulting string=w306:string)  [unwired: 2 in, 1 out]
        n117 = call <vilib>:"Add State(s) to Queue__jki_lib_state_machine.vi"("State(s) in (\"\")"=w310, "State(s) at Back (\"\")"=w306) -> ("States Out"=w309:string)  [unwired: 13 in]
      }
      frame "CMD: Save Chart" {
        n118 = Unbundle By Name(w316) -> ("Indicator Refs.XY Graph"=w315:refnum<vi>)
        n119 = invoke class="XYGraph (strict)" method="Export Data to Excel"(reference=w315, error in=w314) -> (error out=w313:errorcluster)  [unwired: 1 in, 2 out]
      }
    }
  }
  "error out" <- w4
  "reference out" <- "reference in"
